vi "Read PS.vi"(11 "amps?":bool caption="Amps") -> (1 "persistent?":bool caption="Persistent", 2 "rate":dbl caption="Rate", 3 "currentfield":dbl caption="Current Field")   [LabVIEW 2009, in "Magnet.lvclass"]
uses:
  Magnet.lvclass
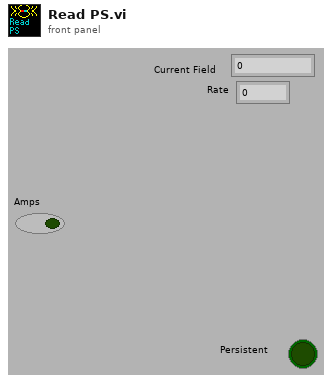
[diagram p1: front panel]
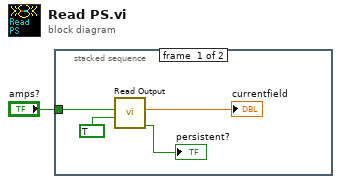
[diagram p0: block diagram]
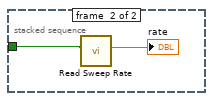
[diagram p2: hidden frame]
diagram:
  n1 = stacked-sequence {
    tunnel: "amps?" -> [w3 w7]
    frame #0 {
      n2 = call "Read Output.vi"("checkpers?"=TRUE, "amp?"=w3) -> ("persistent?"=→"persistent?":bool, "ouput"=→"currentfield":dbl)  [unwired: 4 out]
    }
    frame #1 {
      n3 = call "Read Sweep Rate.vi"("amp?"=w7) -> ("rate"=→"rate":dbl)  [unwired: 6 out]
    }
  }
